vi "标定方式选择对话框.vi"() -> ()   [LabVIEW 2018]
panel:
  in  "空白按钮 4":bool
  in  "空白按钮 3":bool
  in  "空白按钮 2":bool
  in  "空白按钮":bool
  # "标定方式选择对话框"
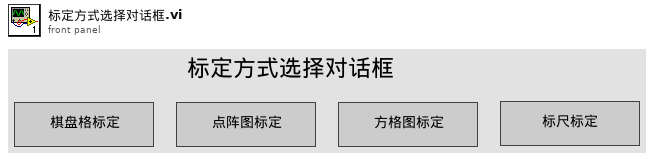
[diagram p1: front panel]
types:
  T1 = enum32{"Invalid", "Standard", "Closed", "Hidden", "Minimized", "Maximized"}
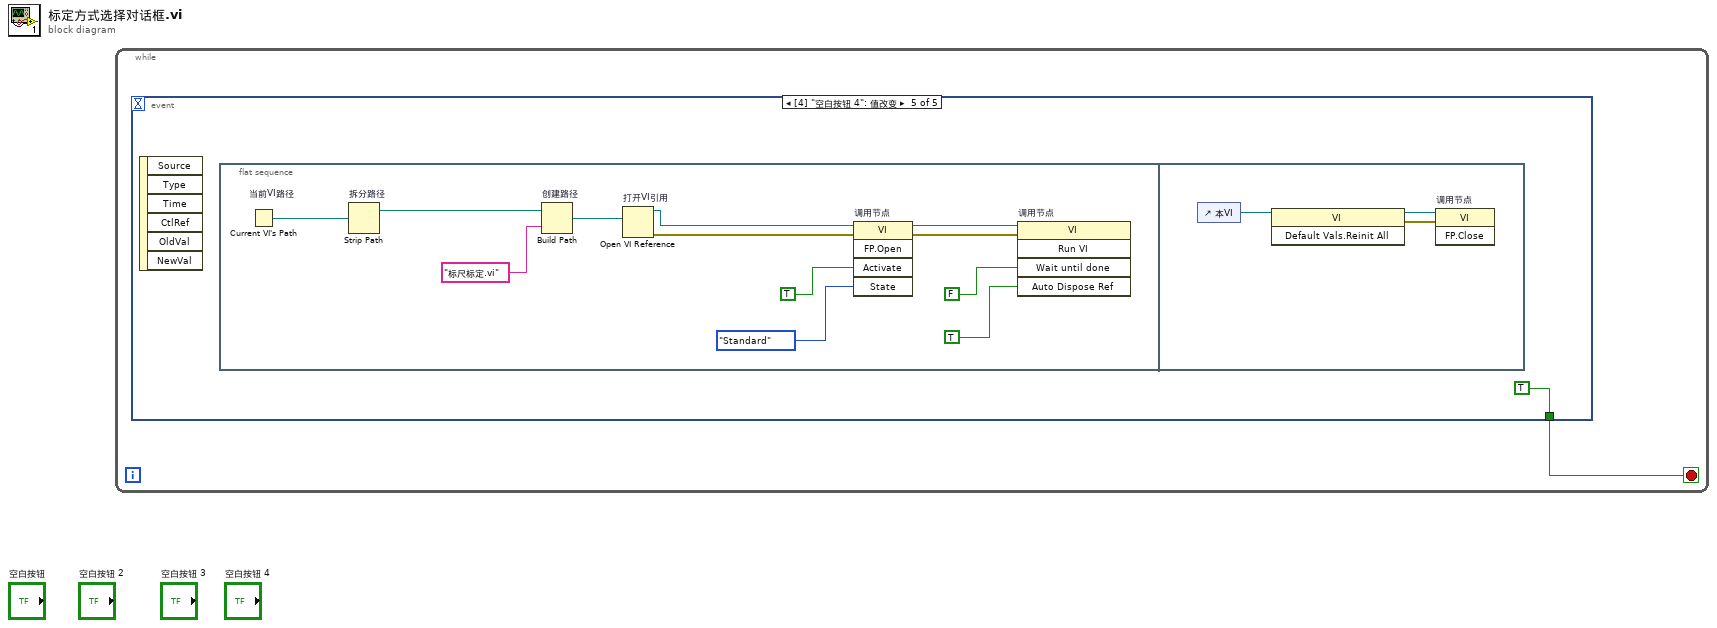
[diagram p0: block diagram]
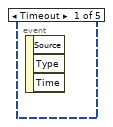
[diagram p2: hidden frame]
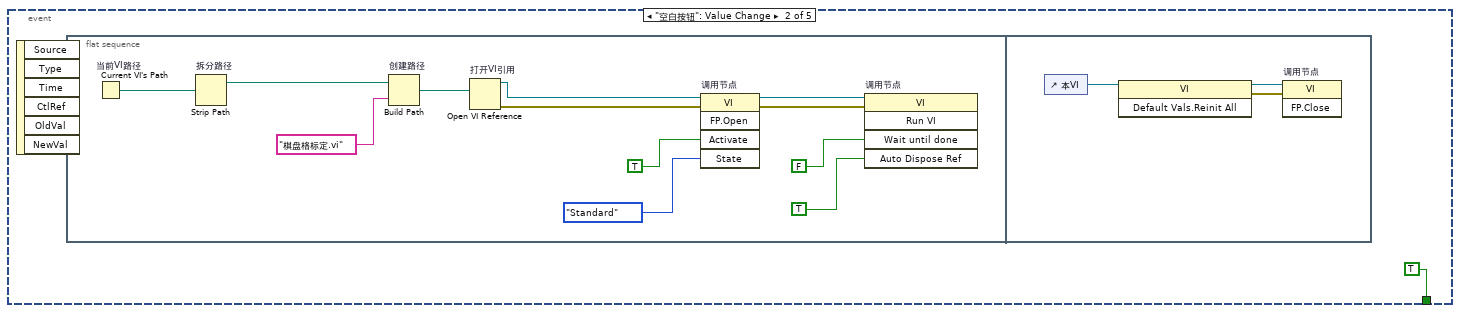
[diagram p3: hidden frame]
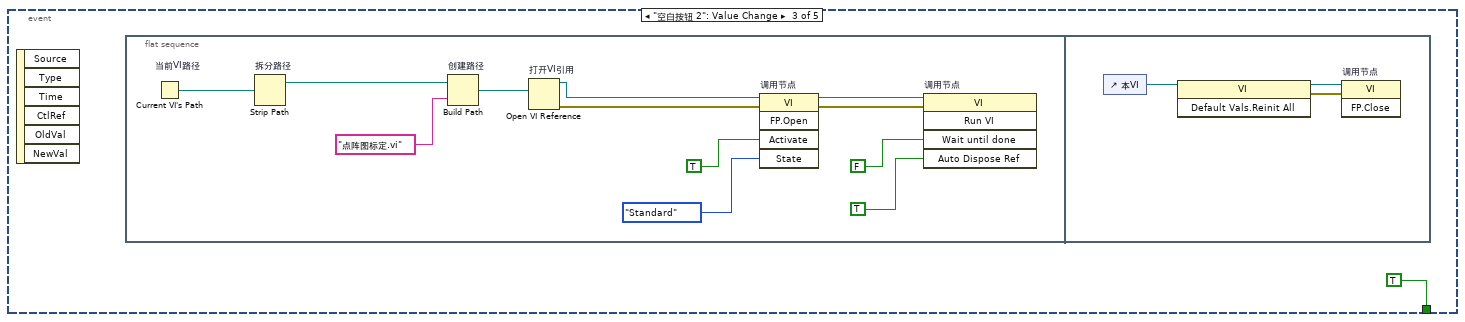
[diagram p4: hidden frame]
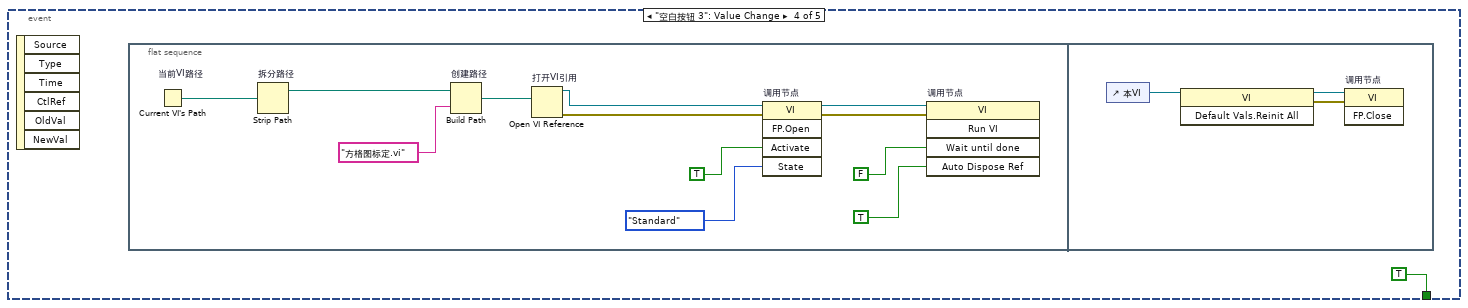
[diagram p5: hidden frame]
diagram:
  n1 = while {
    stop <- w1 stop-if-true
    n2 = event shown="[4] \"空白按钮 4\": 值改变" {
      selector: _ -> [_ _ _ _ _]
      dyn-events: _ -> [_ _ _ _ _]
      timeout: _ -> [_ _ _ _ _]
      tunnel: [_ TRUE TRUE TRUE TRUE] -> w1
      event Timeout {
        n3 = event-data() -> ()  [unwired: 1 in, 3 out]
      }
      event "空白按钮": Value Change {
        n4 = event-data() -> ()  [unwired: 1 in, 6 out]
        n5 = flat-sequence {
          frame #0 {
            n6 = Current VI's Path "当前VI路径"() -> (path=w10:path)
            n7 = Strip Path "拆分路径"(path=w10) -> (stripped path=w14:path)  [unwired: 1 out]
            n8 = Build Path "创建路径"(base path=w14, name or relative path="棋盘格标定.vi" ("名称或相对路径")) -> (appended path=w11:path)
            n9 = Open VI Reference "打开VI引用"(vi path=w11) -> (vi reference=w9:refnum<vi>, error out=w8:errorcluster)  [unwired: 5 in]
            n10 = invoke on="调用节点" class="VI" method="FP.Open"(reference=w9, error in=w8, "Activate"=TRUE ("激活？"), "State"=T1."Standard" ("状态")) -> (reference out=w4:refnum<vi>, error out=w3:errorcluster)  [unwired: 1 in, 3 out]
            n11 = invoke on="调用节点" class="VI" method="Run VI"(reference=w4, error in=w3, "Wait until done"=FALSE ("结束前等待"), "Auto Dispose Ref"=TRUE ("自动销毁引用")) -> ()  [unwired: 1 in, 5 out]
          }
          frame #1 {
            n12 = control-ref of="本VI"() -> (w17:refnum<vi>)
            n13 = invoke class="VI" method="Default Vals.Reinit All"(reference=w17) -> (reference out=w16:refnum<vi>, error out=w15:errorcluster)  [unwired: 2 in, 1 out]
            n14 = invoke on="调用节点" class="VI" method="FP.Close"(reference=w16, error in=w15) -> ()  [unwired: 1 in, 3 out]
          }
        }
      }
      event "空白按钮 2": Value Change {
        n15 = event-data() -> ()  [unwired: 1 in, 6 out]
        n16 = flat-sequence {
          frame #0 {
            n17 = Current VI's Path "当前VI路径"() -> (path=w26:path)
            n18 = Strip Path "拆分路径"(path=w26) -> (stripped path=w30:path)  [unwired: 1 out]
            n19 = Build Path "创建路径"(base path=w30, name or relative path="点阵图标定.vi" ("名称或相对路径")) -> (appended path=w27:path)
            n20 = Open VI Reference "打开VI引用"(vi path=w27) -> (vi reference=w25:refnum<vi>, error out=w24:errorcluster)  [unwired: 5 in]
            n21 = invoke on="调用节点" class="VI" method="FP.Open"(reference=w25, error in=w24, "Activate"=TRUE ("激活？"), "State"=T1."Standard" ("状态")) -> (reference out=w20:refnum<vi>, error out=w19:errorcluster)  [unwired: 1 in, 3 out]
            n22 = invoke on="调用节点" class="VI" method="Run VI"(reference=w20, error in=w19, "Wait until done"=FALSE ("结束前等待"), "Auto Dispose Ref"=TRUE ("自动销毁引用")) -> ()  [unwired: 1 in, 5 out]
          }
          frame #1 {
            n23 = control-ref of="本VI"() -> (w33:refnum<vi>)
            n24 = invoke class="VI" method="Default Vals.Reinit All"(reference=w33) -> (reference out=w32:refnum<vi>, error out=w31:errorcluster)  [unwired: 2 in, 1 out]
            n25 = invoke on="调用节点" class="VI" method="FP.Close"(reference=w32, error in=w31) -> ()  [unwired: 1 in, 3 out]
          }
        }
      }
      event "空白按钮 3": Value Change {
        n26 = event-data() -> ()  [unwired: 1 in, 6 out]
        n27 = flat-sequence {
          frame #0 {
            n28 = Current VI's Path "当前VI路径"() -> (path=w42:path)
            n29 = Strip Path "拆分路径"(path=w42) -> (stripped path=w46:path)  [unwired: 1 out]
            n30 = Build Path "创建路径"(base path=w46, name or relative path="方格图标定.vi" ("名称或相对路径")) -> (appended path=w43:path)
            n31 = Open VI Reference "打开VI引用"(vi path=w43) -> (vi reference=w36:refnum<vi>, error out=w41:errorcluster)  [unwired: 5 in]
            n32 = invoke on="调用节点" class="VI" method="FP.Open"(reference=w36, error in=w41, "Activate"=TRUE ("激活？"), "State"=T1."Standard" ("状态")) -> (reference out=w35:refnum<vi>, error out=w39:errorcluster)  [unwired: 1 in, 3 out]
            n33 = invoke on="调用节点" class="VI" method="Run VI"(reference=w35, error in=w39, "Wait until done"=FALSE ("结束前等待"), "Auto Dispose Ref"=TRUE ("自动销毁引用")) -> ()  [unwired: 1 in, 5 out]
          }
          frame #1 {
            n34 = control-ref of="本VI"() -> (w49:refnum<vi>)
            n35 = invoke class="VI" method="Default Vals.Reinit All"(reference=w49) -> (reference out=w48:refnum<vi>, error out=w47:errorcluster)  [unwired: 2 in, 1 out]
            n36 = invoke on="调用节点" class="VI" method="FP.Close"(reference=w48, error in=w47) -> ()  [unwired: 1 in, 3 out]
          }
        }
      }
      event "空白按钮 4": Value Change {
        n37 = event-data() -> ()  [unwired: 1 in, 6 out]
        n38 = flat-sequence {
          frame #0 {
            n39 = Current VI's Path "当前VI路径"() -> (path=w58:path)
            n40 = Strip Path "拆分路径"(path=w58) -> (stripped path=w62:path)  [unwired: 1 out]
            n41 = Build Path "创建路径"(base path=w62, name or relative path="标尺标定.vi" ("名称或相对路径")) -> (appended path=w59:path)
            n42 = Open VI Reference "打开VI引用"(vi path=w59) -> (vi reference=w52:refnum<vi>, error out=w57:errorcluster)  [unwired: 5 in]
            n43 = invoke on="调用节点" class="VI" method="FP.Open"(reference=w52, error in=w57, "Activate"=TRUE ("激活？"), "State"=T1."Standard" ("状态")) -> (reference out=w51:refnum<vi>, error out=w55:errorcluster)  [unwired: 1 in, 3 out]
            n44 = invoke on="调用节点" class="VI" method="Run VI"(reference=w51, error in=w55, "Wait until done"=FALSE ("结束前等待"), "Auto Dispose Ref"=TRUE ("自动销毁引用")) -> ()  [unwired: 1 in, 5 out]
          }
          frame #1 {
            n45 = control-ref of="本VI"() -> (w65:refnum<vi>)
            n46 = invoke class="VI" method="Default Vals.Reinit All"(reference=w65) -> (reference out=w64:refnum<vi>, error out=w63:errorcluster)  [unwired: 2 in, 1 out]
            n47 = invoke on="调用节点" class="VI" method="FP.Close"(reference=w64, error in=w63) -> ()  [unwired: 1 in, 3 out]
          }
        }
      }
    }
  }
